vi "move.vi"(8 "error in (no error)":errorcluster, 9 "y":i32, 10 "x":i32, 11 "Rectangle in":refnum<class "Rectangle.lvclass">) -> (0 "error out":errorcluster, 3 "Rectangle out":refnum<class "Rectangle.lvclass">)   [LabVIEW 2017, in "Rectangle.lvclass"]
uses:
  Rectangle.lvclass
  Shape Class/Shape.lvclass
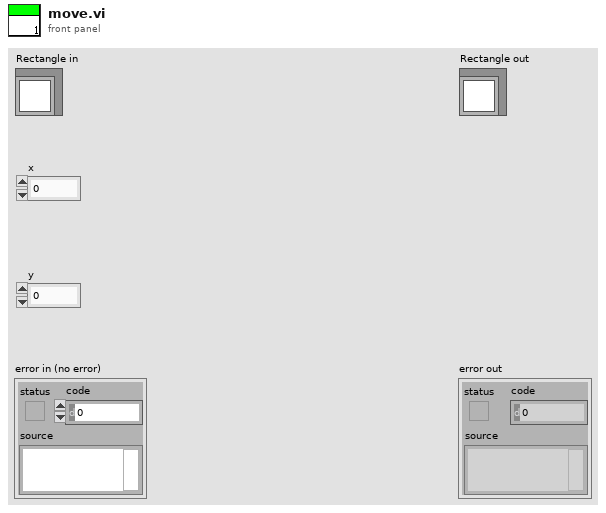
[diagram p1: front panel]
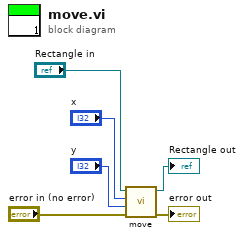
[diagram p0: block diagram]
diagram:
  n1 = call-parent "move.vi"("error in (no error)"="error in (no error)", "y"="y", "x"="x", "Shape in"="Rectangle in") -> ("error out"=→"error out":errorcluster, "Shape out"=→"Rectangle out":refnum<class "Rectangle.lvclass">)  [unwired: 6 in]
